vi "Agilent VNA Set Error Message Mode.vi"(7 "Agilent VNA":T2, 8 "error in (no error)":errorcluster, 10 "Error Message Mode":T1, 11 "VISA Resource Name":refnum<visa-resource-name>) -> (0 "error out":errorcluster, 3 "dup VISA Resource Name":refnum<visa-resource-name>)   [LabVIEW 2011]
doc: "This VI for the HP8753B Network Analyzers reads the stimulus values. Except when performing log sweeps and freq list sweeps, this VI uses the start and stop values and the number of points to calcuate the stimulus values."
uses:
  TypeDefs/Agilent VNA Instrument Info.ctl
  TypeDefs/Agilent VNA Error Message Mode.ctl
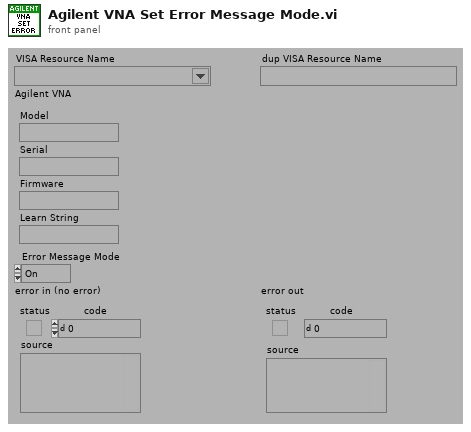
[diagram p1: front panel]
types:
  T1 = typedef "Agilent VNA Error Message Mode.ctl" = enum16{"On", "Off"}
  T2 = typedef "Agilent VNA Instrument Info.ctl" = cluster{"Model":string, "Serial":string, "Firmware":string, "Learn String":string}
  T3 = typedef "Agilent VNA Model.ctl" = enum16{"Not Supported", "8510X", "8719X", "8720X", "8722X", "8753X", "ENA", "PNA", "Field Fox"}
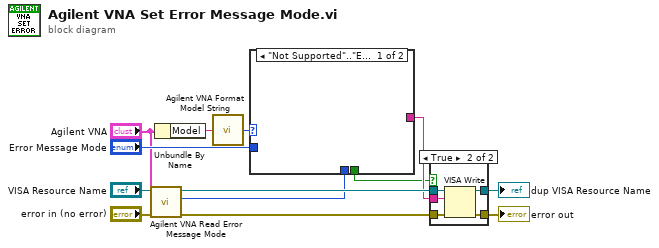
[diagram p0: block diagram]
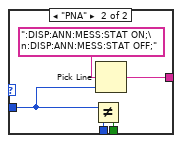
[diagram p2: hidden frame]
diagram:
  n1 = call "Agilent VNA Read Error Message Mode.vi"("Agilent VNA"="Agilent VNA", "error in (no error)"="error in (no error)", "VISA Resource Name"="VISA Resource Name") -> ("error out"=w12:errorcluster, "Error Message Mode"=w4:T1, "dup VISA Resource Name"=w13:refnum<visa-resource-name>)  [unwired: 6 out]
  n2 = Unbundle By Name("Agilent VNA") -> ("Model"=w1:string)
  n3 = call "Agilent VNA Format Model String.vi"("Model"=w1) -> ("Model"=w11:T3)
  n4 = case shown="\"Not Supported\"..\"ENA\", \"Field Fox\"" w11 {
    tunnel: [_ w17] -> w6
    tunnel: "Error Message Mode" -> [_ w16]
    tunnel: w4 -> [_ w15]
    tunnel: [_ w14] -> w3
    frame "Not Supported".."ENA", "Field Fox" {
    }
    frame "PNA" {
      n5 = Not Equal?(x=w16, y=w15) -> (x != y?=w14:bool)
      n6 = Pick Line(multi-line string=":DISP:ANN:MESS:STAT ON;\n:DISP:ANN:MESS:STAT OFF;", line index=w16) -> (output string=w17:string)  [unwired: 1 out]
    }
  }
  n7 = case shown="True" w3 {
    tunnel: [w19 w25] -> w7
    tunnel: [w20 w24] -> w8
    tunnel: w6 -> [_ w23]
    tunnel: w13 -> [w20 w22]
    tunnel: w12 -> [w19 w21]
    frame False {
    }
    frame True {
      n8 = VISA Write(VISA resource name=w22, write buffer=w23, error in (no error)=w21) -> (VISA resource name out=w24:refnum<visa-resource-name>, error out=w25:errorcluster)  [unwired: 1 out]
    }
  }
  "dup VISA Resource Name" <- w8
  "error out" <- w7
